vi "FlagInitialized.vi"(10 "User Events Reference":T1, 11 "InterfaceRef":T2) -> (3 "InterfaceRefOut":T2)   [LabVIEW 2017, in "ImageAcquisitionLibrary.lvlib"]
uses:
  ImageAcquisitionProgram/ImageAcquisitionLibrary/ImageAcquisitionLibrary.lvlib
  InterfaceReferences.ctl
  EventsReference.ctl
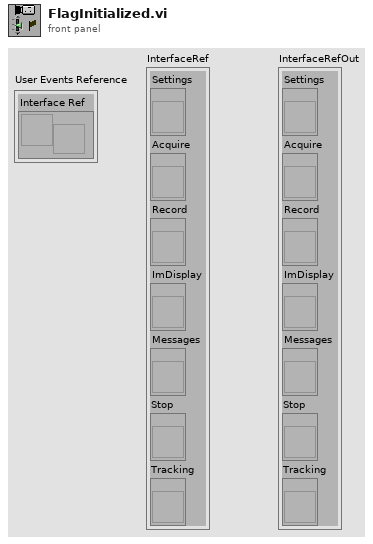
[diagram p1: front panel]
types:
  T1 = typedef "ImageAcquisitionLibrary.lvlib/EventsReference.ctl" = cluster{"Interface Ref":refnum<user-event>}
  T2 = typedef "ImageAcquisitionLibrary.lvlib/InterfaceReferences.ctl" = cluster{"Settings":refnum<vi>, "Acquire":refnum<vi>, "Record":refnum<vi>, "ImDisplay":refnum<vi>, "Messages":refnum<vi>, "Stop":refnum<vi>, "Tracking":refnum<vi>}
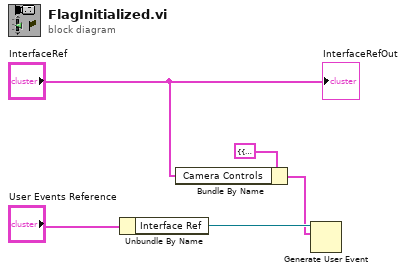
[diagram p0: block diagram]
diagram:
  n1 = Unbundle By Name("User Events Reference") -> ("Interface Ref"=w5:refnum<user-event>)
  n2 = Bundle By Name(cluster=cluster{"Camera Controls":T2} {"Camera Controls"={"Settings"=refnum, "Acquire"=refnum, "Record"=refnum, "ImDisplay"=refnum, "Messages"=refnum, "Stop"=refnum, "Tracking"=refnum}} ("event data"), "Camera Controls"="InterfaceRef") -> (w1:cluster{"Camera Controls":T2})
  n3 = Generate User Event(user event=w5, event data cluster=w1) -> ()  [unwired: 2 in, 2 out]
  "InterfaceRefOut" <- "InterfaceRef"
